vi "Create Client.vi"(8 "error in":errorcluster, 11 "cluster id":string) -> (0 "error out":errorcluster, 3 "grpc client id":T1)   [LabVIEW 2020, in "MeasurementServerTests.lvlib"]
uses:
  MeasurementServerTests.lvlib
  <vilib>/gRPC/LabVIEW gRPC Library/Shared/grpcId.ctl
  Runtime/MeasurementLink Discovery Client/RPC Messages/ni_measurementlink_discovery_v1_ResolveServiceRequest.ctl
  Runtime/MeasurementLink Discovery V1/MeasurementLink Discovery V1.lvlib
  Runtime/MeasurementLink Discovery Client/MeasurementLink Discovery Client.lvlib
  Runtime/MeasurementLink Pin Map Client/MeasurementLink Pin Map Client.lvlib
  <vilib>/gRPC/LabVIEW gRPC Library/grpc-lvsupport-release.lvlib
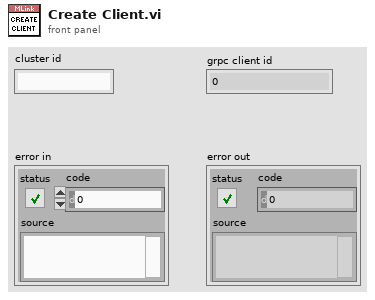
[diagram p1: front panel]
types:
  T1 = typedef "grpc-lvsupport-release.lvlib/grpcId.ctl" = u64
  T2 = typedef "MeasurementLink Discovery Client.lvlib/ni_measurementlink_discovery_v1_ResolveServiceRequest.ctl" = cluster{"provided_interface":string, "service_class":string}
  T3 = typedef "MeasurementLink Discovery Client.lvlib/ni_measurementlink_discovery_v1_ServiceLocation.ctl" = cluster{"location":string, "insecure_port":string, "ssl_authenticated_port":string}
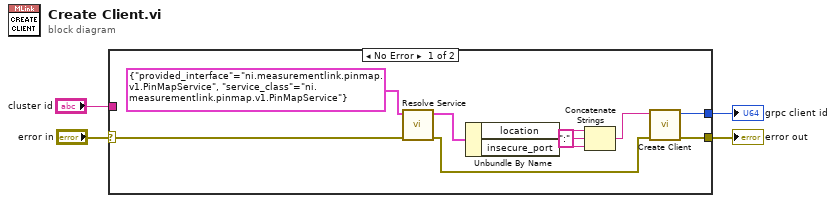
[diagram p0: block diagram]
diagram:
  n1 = case shown="No Error" "error in" {
    selector: "error in" -> [w12 w15]
    tunnel: [w11 _] -> w3
    tunnel: [w10 w15] -> w2
    tunnel: "cluster id" -> [_ _]
    frame No Error {
      n2 = call "Resolve Service.vi"("error in"=w12, "request data"=T2 {"provided_interface"="ni.measurementlink.pinmap.v1.PinMapService", "service_class"="ni.measurementlink.pinmap.v1.PinMapService"}) -> ("error out"=w13:errorcluster, "response data"=w14:T3)  [unwired: 8 in]
      n3 = Unbundle By Name(w14) -> ("location"=w6:string, "insecure_port"=w7:string)
      n4 = Concatenate Strings(w6, ":" ("string"), w7) -> (w9:string)
      n5 = call "Create Client.vi"("error in"=w13, "address"=w9) -> ("error out"=w10:errorcluster, "gRPC ID Out"=w11:T1)  [unwired: 8 in]
    }
    frame Error {
    }
  }
  "grpc client id" <- w3
  "error out" <- w2
